vi "Main.vi"() -> ()   [LabVIEW 2020]
doc: "This template is for the Queued Message Handler design pattern.\n\nThe Event Handling Loop generates messages based on user interface actions.\n\nThe Message Handling Loop processes messages generated by the Event Handling Loop, or by other messages. The messages are string values, so new messages can be added easily to the Message Cases case structure in the Message Handling Loop. Each message cluster can also provide an optional value for Message Data, which is a variant that can be converted to whatever message-specific data is required."
uses:
  Snake/Type Defs/Direction.ctl
  Snake/Type Defs/Coordinates.ctl
  Game Board/Game Board.lvclass/Game Board.ctl
  Game Board/Generate.vi
  Snake/tail.get.vi
  Game Board/board.replace_pixel.vi
  Snake/Snake.lvclass
  Game Board/Game Board.lvclass
  Fruit/Fruit.lvclass
panel:
  out "Score":u32
  out "Board":u32[][](array[colorbox])
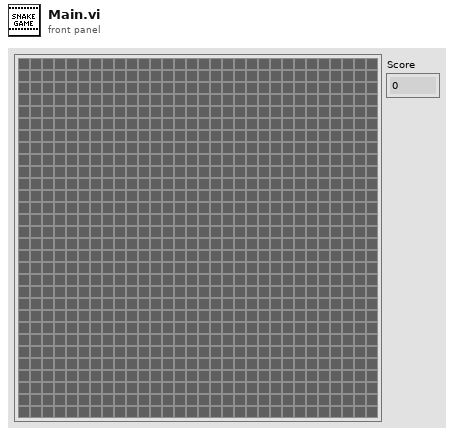
[diagram p1: front panel]
types:
  T1 = typedef "Coordinates.ctl" = cluster{"X":i32, "Y":i32}
  T2 = typedef "Direction.ctl" = enum16{"Up", "Down", "Left", "Right"}
  T3 = typedef "eventvkey.ctl" = enum16{"ASCII", "Enter", "Return", "Shift", "Ctrl", "Alt", "Cmd", "Opt", "Caps", "NumLock", "Clear", "Break", "Up", "Down", "Left", "Right", "Insert", "Delete", "Home", "End", "PageUp", "PageDown", "Escape", "Help", "Pause", "ScrollLock", "F1", "F2", "F3", "F4", "F5", "F6", "F7", "F8", "F9", "F10", "F11", "F12", "F13", "F14", "F15", "F16", "F17", "F18", "F19", "F20", "F21", "F22", "F23", "F24", "Play", "VolumeUp", "VolumeDown", "Mute", "Two Byte Char"}
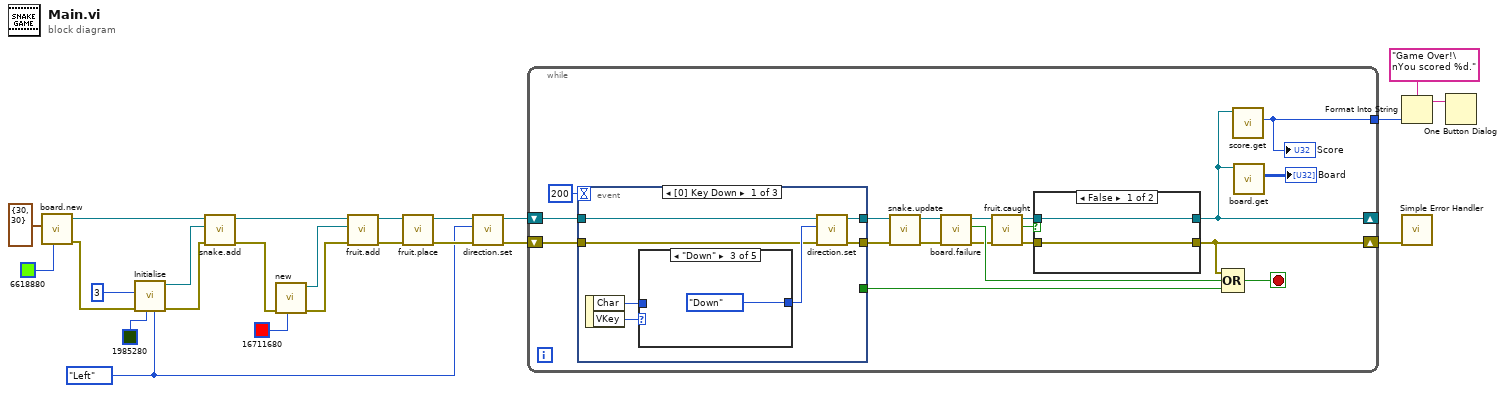
[diagram p0: block diagram]
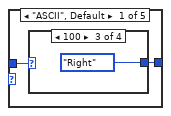
[diagram p2: hidden frame]
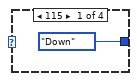
[diagram p3: hidden frame]
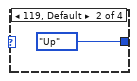
[diagram p4: hidden frame]
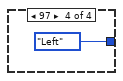
[diagram p5: hidden frame]
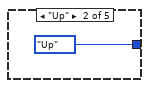
[diagram p6: hidden frame]
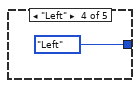
[diagram p7: hidden frame]
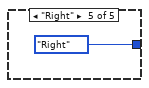
[diagram p8: hidden frame]
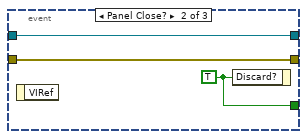
[diagram p9: hidden frame]
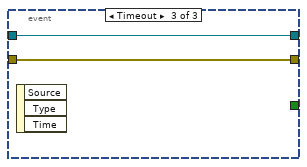
[diagram p10: hidden frame]
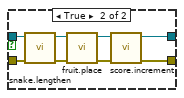
[diagram p11: hidden frame]
diagram:
  w2 = Direction."Left" ("Direction")
  n1 = call "board.new.vi"("Color Box"=u32 6618880, "Grid Size"=T1 {"X"=30, "Y"=30}) -> ("error out"=w13:errorcluster, "Game Board out"=w20:refnum<class "Game Board.lvclass">)  [unwired: 8 in]
  n2 = call "Initialise.vi"("Direction"=w2, "Snake Colour"=u32 1985280, "error in (no error)"=w13, "Starting Elements"=3) -> ("error out"=w14:errorcluster, "Snake out"=w19:refnum<class "Snake.lvclass">)  [unwired: 6 in]
  n3 = call "snake.add.vi"("error in (no error)"=w14, "Snake in"=w19, "Game Board in"=w20) -> ("error out"=w15:errorcluster, "Game Board out"=w16:refnum<class "Game Board.lvclass">)  [unwired: 7 in]
  n4 = call "new.vi"("Color Box"=u32 16711680, "error in (no error)"=w15) -> ("error out"=w12:errorcluster, "Fruit out"=w17:refnum<class "Fruit.lvclass">)  [unwired: 8 in]
  n5 = call "fruit.add.vi"("error in (no error)"=w12, "Fruit.lvclass"=w17, "Game Board in"=w16) -> ("error out"=w10:errorcluster, "Game Board out"=w11:refnum<class "Game Board.lvclass">)  [unwired: 7 in]
  n6 = call "fruit.place.vi"("error in (no error)"=w10, "Game Board in"=w11) -> ("error out"=w5:errorcluster, "Game Board out"=w6:refnum<class "Game Board.lvclass">)  [unwired: 8 in]
  n7 = call "direction.set.vi"("error in (no error)"=w5, "Direction"=w2, "Game Board in"=w6) -> ("error out"=w4:errorcluster, "Game Board out"=w3:refnum<class "Game Board.lvclass">)  [unwired: 7 in]
  n8 = while {
    shift-right: [w37] -> _
    shift-left: w3 -> [w32]
    tunnel: [w35] -> w9
    shift-right: [w26] -> w1
    shift-left: w4 -> [w31]
    stop <- w27 stop-if-true
    n9 = event shown="[0] Key Down" {
      selector: _ -> [_ _ _]
      dyn-events: _ -> [_ _ _]
      timeout: 200 -> [_ _ _]
      tunnel: [_ w63 _] -> w29
      tunnel: [w48 w62 w64] -> w34
      tunnel: [w47 w61 w65] -> w33
      tunnel: w32 -> [w45 w61 w65]
      tunnel: w31 -> [w44 w62 w64]
      event Key Down {
        n10 = event-data() -> ("Char"=w50:i16, "VKey"=w49:T3)  [unwired: 1 in]
        n11 = case shown="\"Down\"" w49 {
          tunnel: w50 -> [w52 _ _ _ _]
          tunnel: [w51 Direction."Up" ("Direction") Direction."Down" ("Direction") Direction."Left" ("Direction") Direction."Right" ("Direction")] -> w46
          frame "ASCII", Default {
            n12 = case shown="100" w52 {
              tunnel: [Direction."Down" ("Direction") Direction."Up" ("Direction") Direction."Right" ("Direction") Direction."Left" ("Direction")] -> w51
              frame 115 {
              }
              frame 119, Default {
              }
              frame 100 {
              }
              frame 97 {
              }
            }
          }
          frame "Up" {
          }
          frame "Down" {
          }
          frame "Left" {
          }
          frame "Right" {
          }
        }
        n13 = call "direction.set.vi"("error in (no error)"=w44, "Direction"=w46, "Game Board in"=w45) -> ("error out"=w48:errorcluster, "Game Board out"=w47:refnum<class "Game Board.lvclass">)  [unwired: 7 in]
      }
      event Panel Close? {
        w63 = TRUE ("Discard?")
        n14 = event-data() -> ()  [unwired: 1 in, 1 out]
        n15 = event-data("Discard?"=w63) -> ()  [unwired: 1 in, 1 out]
      }
      event Timeout {
        n16 = event-data() -> ()  [unwired: 1 in, 3 out]
      }
    }
    n17 = call "snake.update.vi"("error in (no error)"=w34, "Game Board in"=w33) -> ("error out"=w41:errorcluster, "Game Board out"=w42:refnum<class "Game Board.lvclass">)  [unwired: 8 in]
    n18 = call "board.failure.vi"("error in (no error)"=w41, "Game Board in"=w42) -> ("error out"=w28:errorcluster, "Fail"=w30:bool, "Game Board out"=w40:refnum<class "Game Board.lvclass">)  [unwired: 7 in]
    n19 = call "fruit.caught.vi"("error in (no error)"=w28, "Game Board in"=w40) -> ("error out"=w38:errorcluster, "Fruit Caught"=w36:bool, "Game Board out"=w39:refnum<class "Game Board.lvclass">)  [unwired: 7 in]
    n20 = case shown="False" w36 {
      tunnel: w39 -> [w67 w75]
      tunnel: w38 -> [w66 w74]
      tunnel: [w67 w69] -> w37
      tunnel: [w66 w68] -> w26
      frame False {
      }
      frame True {
        n21 = call "snake.lengthen.vi"("error in (no error)"=w74, "Game Board in"=w75) -> ("error out"=w72:errorcluster, "Game Board out"=w73:refnum<class "Game Board.lvclass">)  [unwired: 8 in]
        n22 = call "fruit.place.vi"("error in (no error)"=w72, "Game Board in"=w73) -> ("error out"=w70:errorcluster, "Game Board out"=w71:refnum<class "Game Board.lvclass">)  [unwired: 8 in]
        n23 = call "score.increment.vi"("error in (no error)"=w70, "Game Board in"=w71) -> ("error out"=w68:errorcluster, "Game Board out"=w69:refnum<class "Game Board.lvclass">)  [unwired: 8 in]
      }
    }
    n24 = Compound Arithmetic op=OR(w26, w30, w29) -> (w27:bool)
    n25 = call "score.get.vi"("Game Board in"=w37) -> ("Score"=w35:u32)  [unwired: 10 in]
    "Score" <- w35
    n26 = call "board.get.vi"("Game Board in"=w37) -> ("Game Board"=→"Board":u32[][])  [unwired: 10 in]
  }
  n27 = Format Into String(format string="Game Over!\nYou scored %d.", w9) -> (resulting string=w8:string)  [unwired: 2 in, 1 out]
  n28 = call <vilib>:"Simple Error Handler.vi"("error in (no error)"=w1) -> ()  [unwired: 4 in, 5 out]
  n29 = One Button Dialog(message=w8) -> ()  [unwired: 1 in, 1 out]
